vi "IBM4_PWM.vi"(0 "COM resource in":refnum<visa-resource-name>="COM9", 2 "PWM(%)":dbl=50.0, 3 "error in":errorcluster) -> (7 "COM resource out":refnum<visa-resource-name>="COM9", 10 "error out":errorcluster)   [LabVIEW 2023, in "IBM4.lvlib"]
doc: "This VI interfaces with the IBM4 to set a pulse wave modulated (PWM) output signal.\nThe output Pin# must be: 5,7,9,10-13.\nThe PWM output must be between 0 and 100, and is a floating point value."
uses:
  <instrlib>/IBM4/IBM4.lvlib
panel:
  out "read buffer":string="PWMset 13 = 10.0 \r\n"
  in  "Pin#":i32=9
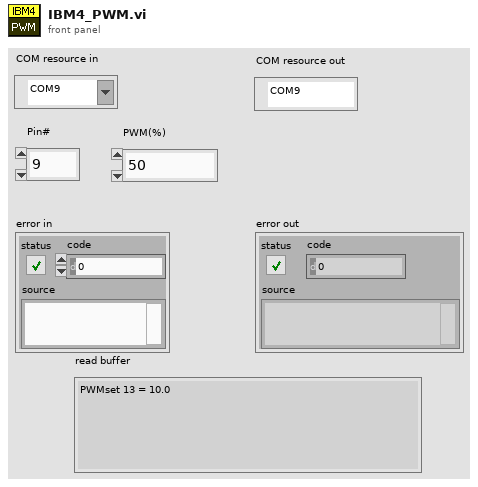
[diagram p1: front panel]
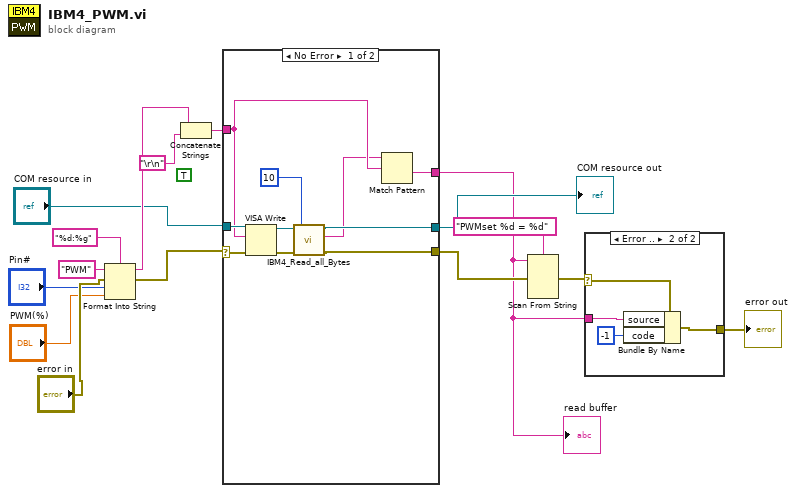
[diagram p0: block diagram]
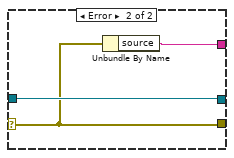
[diagram p3: hidden frame]
diagram:
  (unwired) TRUE ("Enable Termination\nChar (T)")
  n1 = Format Into String(format string="%d:%g", initial string="PWM", error in="error in", "Pin#", "PWM(%)") -> (resulting string=w7:string, error out=w1:errorcluster)
  n2 = Concatenate Strings(w7, "\r\n") -> (w6:string)
  n3 = case shown="No Error" w1 {
    selector: w1 -> [w23 w27]
    tunnel: "COM resource in" -> [w26 w29]
    tunnel: [w19 w27] -> w10
    tunnel: [w25 w28] -> w3
    tunnel: w6 -> [w24 _]
    tunnel: [w20 w29] -> w11
    frame No Error {
      n4 = VISA Write(VISA resource name=w26, write buffer=w24, error in (no error)=w23) -> (VISA resource name out=w22:refnum<visa-resource-name>, error out=w21:errorcluster)  [unwired: 1 out]
      n5 = call <instrlib>:"IBM4_Read_all_Bytes.vi"("error in (no error)"=w21, "milliseconds to wait"=u32 10, "VISA Refnum in"=w22) -> ("error out"=w19:errorcluster, "String"=w18:string, "VISA Refnum out"=w20:refnum<visa-resource-name>)  [unwired: 2 in]
      n6 = Match Pattern(string=w18, regular expression=w24) -> (after substring=w25:string)  [unwired: 1 in, 3 out]
    }
    frame Error {
      n7 = Unbundle By Name(w27) -> ("source"=w28:string)
    }
  }
  "COM resource out" <- w11
  "read buffer" <- w3
  n8 = Scan From String(format string="PWMset %d = %d", input string=w3, error in=w10) -> (error out=w5:errorcluster)  [unwired: 5 in, 2 out]
  n9 = case shown="Error .." w5 {
    selector: w5 -> [w30 w34]
    tunnel: [w30 w32] -> w4
    tunnel: w3 -> [_ w33]
    frame No Error {
    }
    frame Error {
      n10 = Bundle By Name(cluster=w34, "source"=w33, "code"=-1) -> (w32:errorcluster)
    }
  }
  "error out" <- w4
